vi "Points_to_Circle_Parameters.vi"(9 "Arc End point":dbl[](array[numeric]), 10 "Arc Start point":dbl[](array[numeric])) -> (0 "Center point":T1, 1 "Radius":dbl, 2 "Center Deg":dbl, 3 "Start Deg":dbl)   [LabVIEW 2014]
doc: "在二维图中画弧线"
uses:
  <vilib>/Analysis/_algsub.llb/Real Vector Norm.vi
  <vilib>/Analysis/baseanly.llb/Real Dot Product.vi
  <vilib>/Analysis/NI_AALPro.lvlib
  <vilib>/Analysis/NI_AALBase.lvlib
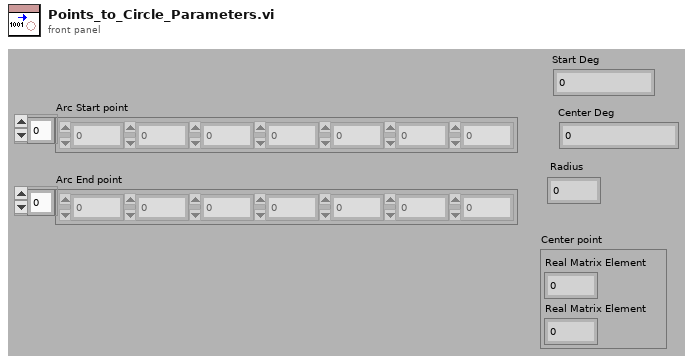
[diagram p1: front panel]
types:
  T1 = cluster{"Real Matrix Element":dbl, "Real Matrix Element":dbl}
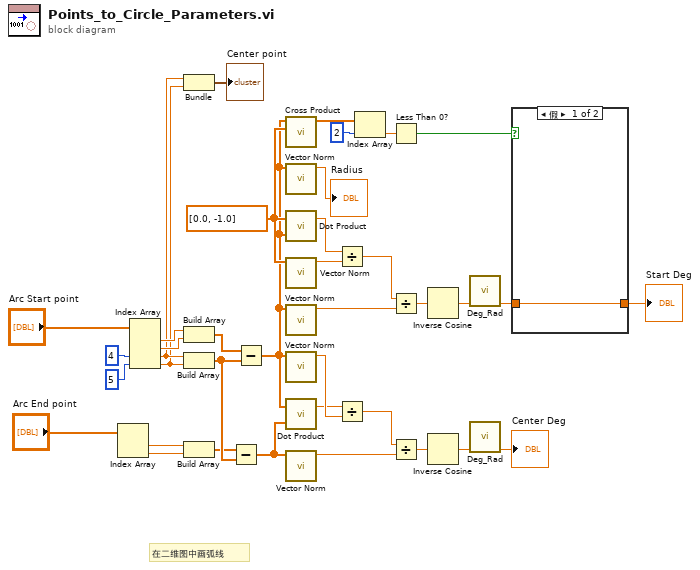
[diagram p0: block diagram]
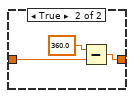
[diagram p2: hidden frame]
diagram:
  w8 = dbl[] [0.0, -1.0] ("Input Vector")
  # "在二维图中画弧线"
  n1 = Index Array(array="Arc End point") -> (element #1=w33:dbl, element #2=w32:dbl)  [unwired: 2 in]
  n2 = Index Array(array="Arc Start point", index #3=4 ("索引"), index #4=5 ("索引")) -> (element #1=w35:dbl, element #2=w34:dbl, element #3=w31:dbl, element #4=w30:dbl)  [unwired: 2 in]
  n3 = Bundle("Real Matrix Element"=w31, "Real Matrix Element"=w30) -> (→"Center point":T1)  [unwired: 1 in]
  n4 = Build Array(w35, w34) -> (w14:dbl[])
  n5 = Build Array(w31, w30) -> (w13:dbl[])
  n6 = Build Array(w33, w32) -> (w12:dbl[])
  n7 = Subtract(x=w12, y=w13) -> (x-y=w11:dbl[])
  n8 = Subtract(x=w14, y=w13) -> (x-y=w7:dbl[])
  n9 = call <vilib>:"Cross Product.vi"("B Vector"=w8, "A Vector"=w7) -> ("Cross Product"=w6:dbl[])  [unwired: 8 in, 1 out]
  n10 = call-poly <vilib>:"Vector Norm.vi"("Input Vector"=w7) -> ("norm"=→"Radius":dbl)  [unwired: 9 in, 1 out]
  n11 = call-poly <vilib>:"Dot Product.vi"("Y Vector"=w7, "X Vector"=w8) -> ("X * Y"=w19:dbl)  [unwired: 1 out]
  n12 = call-poly <vilib>:"Vector Norm.vi"("Input Vector"=w8) -> ("norm"=w18:dbl)  [unwired: 9 in, 1 out]
  n13 = call-poly <vilib>:"Vector Norm.vi"("Input Vector"=w7) -> ("norm"=w16:dbl)  [unwired: 9 in, 1 out]
  n14 = call-poly <vilib>:"Vector Norm.vi"("Input Vector"=w7) -> ("norm"=w24:dbl)  [unwired: 9 in, 1 out]
  n15 = call-poly <vilib>:"Dot Product.vi"("Y Vector"=w11, "X Vector"=w7) -> ("X * Y"=w23:dbl)  [unwired: 1 out]
  n16 = call-poly <vilib>:"Vector Norm.vi"("Input Vector"=w11) -> ("norm"=w26:dbl)  [unwired: 9 in, 1 out]
  n17 = Divide(x=w19, y=w18) -> (x/y=w17:dbl)
  n18 = Divide(x=w23, y=w24) -> (x/y=w25:dbl)
  n19 = Index Array(array=w6, index=2 ("索引")) -> (element=w4:dbl)
  n20 = Less Than 0?(x=w4) -> (x < 0?=w3:bool)
  n21 = Divide(x=w17, y=w16) -> (x/y=w15:dbl)
  n22 = Divide(x=w25, y=w26) -> (x/y=w27:dbl)
  n23 = Inverse Cosine(1:w15) -> (0:w20:dbl)
  n24 = Inverse Cosine(1:w27) -> (0:w22:dbl)
  n25 = call "Deg_Rad.vi"("Rad"=w20) -> ("Deg"=w2:dbl)  [unwired: 9 in, 1 out]
  n26 = call "Deg_Rad.vi"("Rad"=w22) -> ("Deg"=→"Center Deg":dbl)  [unwired: 9 in, 1 out]
  n27 = case shown="假" w3 {
    tunnel: w2 -> [w38 w41]
    tunnel: [w38 w39] -> w1
    frame False {
    }
    frame True {
      n28 = Subtract(x=360.0, y=w41) -> (x-y=w39:dbl)
    }
  }
  "Start Deg" <- w1
